vi "ExCircAccumNframeBin2x.vi"() -> ()   [LabVIEW 2010]
panel:
  in  "Number of software acuums":u32=1 min=1 step=1
  in  "Timing Mode":u32(ring)=1 items=["N/A", "Timed Mode/Free run", "Trigger First (only PM)", "Strobed/Ext Sync", "Bulb Mode (PM only)", "Variable Timed mode (PM only)", "Flash Mode (only some PM)"]
  in  "Number of Images":u32=1 min=1 step=1
  in  "Intensifier":bool
  in  "Temperature":dbl=-10.0 format="%.2f"
  in  "Exposure":dbl min=0.0 step=0.001 format="%.3f"
  out "error out":errorcluster
  in  "error in (no error)":errorcluster
  # "ExCircAccumNframeBin2x:\nThis example collects, displays, and saves in \na .spe file the number of images selected. This\nexample also shows how to store frames using\nsoftware accumulation (addtion). This example\n requires the camera have circular buffers \ncapability."
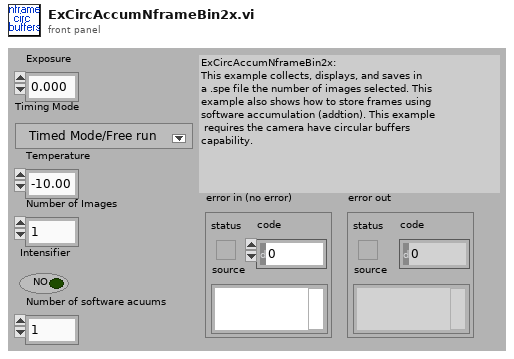
[diagram p1: front panel]
types:
  T1 = cluster{"acquire focus mode":u32, "Exposure":dbl, "Number of Images":u32, "Number of software acuums":u32}
  T2 = cluster{"Camera Handle":u32, "Pulser Handle":u32, "File Handle":u32, "Display Handle":u32, "Image Handle":u32}
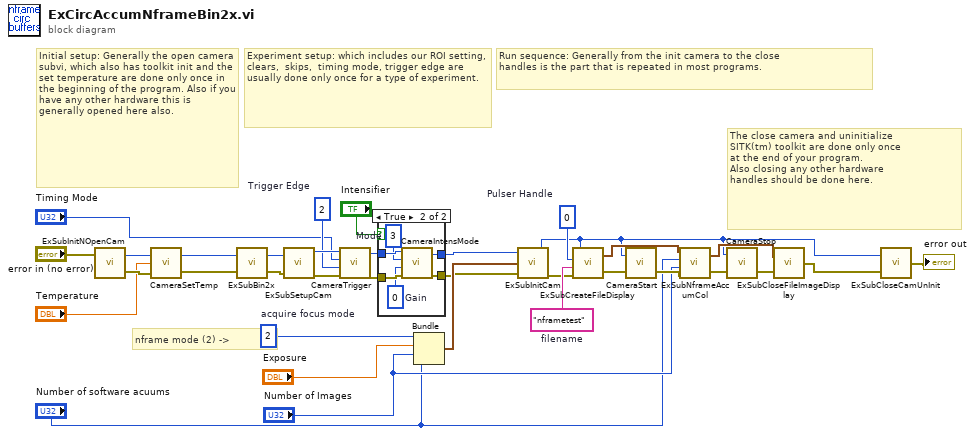
[diagram p0: block diagram]
diagram:
  w24 = u32 0  # Pulser Handle
  w25 = u32 2  # Trigger Edge
  w26 = u32 2  # acquire focus mode
  w34 = "nframetest"  # filename
  # "The close camera and uninitialize\nSITK(tm) toolkit are done only once\nat the end of your program.\nAlso closing any other hardware \nhandles should be done here."
  # "Run sequence: Generally from the init camera to the close \nhandles is the part that is repeated in most programs."
  # "Experiment setup: which includes our ROI setting, clears,  skips,  timing mode, trigger edge are usually done only once for a type of experiment."
  # "Initial setup: Generally the open camera subvi, which also has toolkit init and the set temperature are done only once in the beginning of the program. Also if you have any other hardware this is generally opened here also."
  # "nframe mode (2) ->"
  n1 = call "ExSubInitNOpenCam.vi"("error in (no error)"="error in (no error)") -> ("Camera Handle"=w13:u32, "error out"=w12:errorcluster)
  n2 = call <userlib>:"CameraSetTemp.vi"("error in (no error)"=w12, "Temperature"="Temperature", "Camera Handle"=w13) -> ("error out"=w15:errorcluster, "Camera Handle"=w14:u32)
  n3 = call "ExSubBin2x.vi"("error in (no error)"=w15, "Camera Handle"=w14) -> ("error out"=w9:errorcluster, "Camera Handle"=w10:u32)
  n4 = call "ExSubSetupCam.vi"("error in (no error)"=w9, "Camera Handle"=w10) -> ("error out"=w28:errorcluster, "Camera Handle"=w29:u32)
  n5 = call <userlib>:"CameraTrigger.vi"("error in"=w28, "Trigger Edge"=w25, "Timing Mode"="Timing Mode", "Camera Handle"=w29) -> ("error out"=w21:errorcluster, "Camera Handle"=w23:u32)
  n6 = case shown="True" "Intensifier" {
    tunnel: w23 -> [w36 w42]
    tunnel: [w36 w41] -> w22
    tunnel: w21 -> [w35 w40]
    tunnel: [w35 w39] -> w20
    frame False {
    }
    frame True {
      w37 = u32 0  # Gain
      w38 = u32 3  # Mode
      n7 = call <userlib>:"CameraIntensMode.vi"("error in"=w40, "Intensifier Gain"=w37, "Mode"=w38, "Camera Handle"=w42) -> ("error out"=w39:errorcluster, "Camera Handle"=w41:u32)
    }
  }
  n8 = Bundle("acquire focus mode"=w26, "Exposure"="Exposure", "Number of Images"="Number of Images", "Number of software acuums"="Number of software acuums") -> (w31:T1)  [unwired: 1 in]
  n9 = call "ExSubInitCam.vi"("error in (no error)"=w20, "Camera Information"=w31, "Camera Handle"=w22) -> ("error out"=w30:errorcluster, "Camera Handle"=w4:u32)
  n10 = call "ExSubCreateFileDisplay.vi"("error in (no error)"=w30, "File and Display Name"=w34, "Pulser Handle"=w24, "Camera Handle"=w4) -> ("error out"=w27:errorcluster, "Handles Out"=w18:T2)
  n11 = call <userlib>:"CameraStart.vi"("error in"=w27, "Camera Handle"=w4) -> ("error out"=w17:errorcluster)  [unwired: 1 out]
  n12 = call "ExSubNframeAccumCol.vi"("error in (no error)"=w17, "Number of Images"="Number of Images", "Software accumulations"="Number of software acuums", "Handle Cluster"=w18) -> ("error out"=w8:errorcluster, "Handle Cluster"=w7:T2)
  n13 = call <userlib>:"CameraStop.vi"("error in"=w8, "Camera Handle"=w4) -> ("error out"=w6:errorcluster)  [unwired: 1 out]
  n14 = call "ExSubCloseFileImageDisplay.vi"("error in (no error)"=w6, "Handles In"=w7) -> ("error out"=w5:errorcluster)
  n15 = call "ExSubCloseCamUnInit.vi"("error in (no error)"=w5, "Camera Handle"=w4) -> ("error out"=→"error out":errorcluster)
